vi "17O std simple.vi"(8 "error in":errorcluster) -> (0 "error out":errorcluster)   [LabVIEW 2016]
uses:
  controls/data control cluster.ctl
panel:
  out "transposed array":dbl[][](array[numeric])
  in  "number of sequence to combine":dbl=1.0
  out "Array":dbl[][](array[numeric])
  out "output cluster":T1
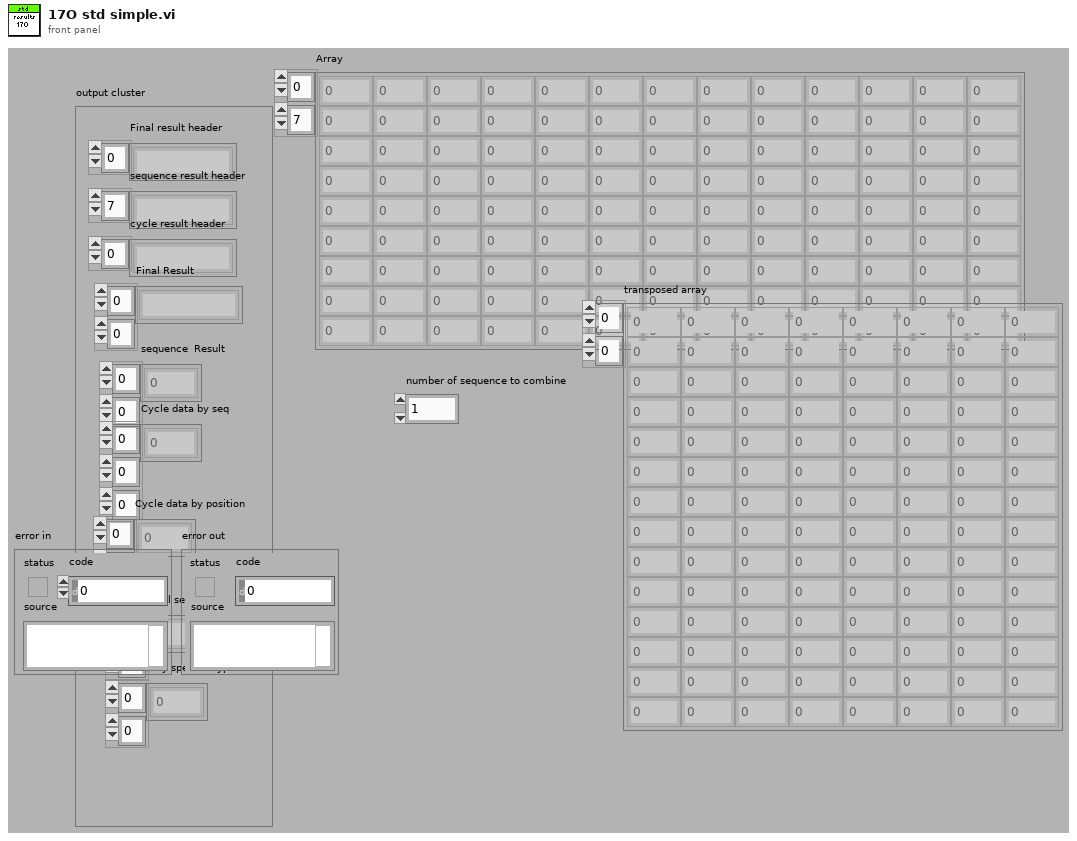
[diagram p1: front panel]
types:
  T1 = typedef "data control cluster.ctl" = cluster{"Final result header":string[], "sequence result header":string[], "cycle result header ":string[], "Final Result":string[][], "sequence  Result":dbl[][], "Cycle data by seq":dbl[][][], "Cycle data by position":dbl[][][], "Final seq  Result":dbl[][], "only specific type":dbl[][]}
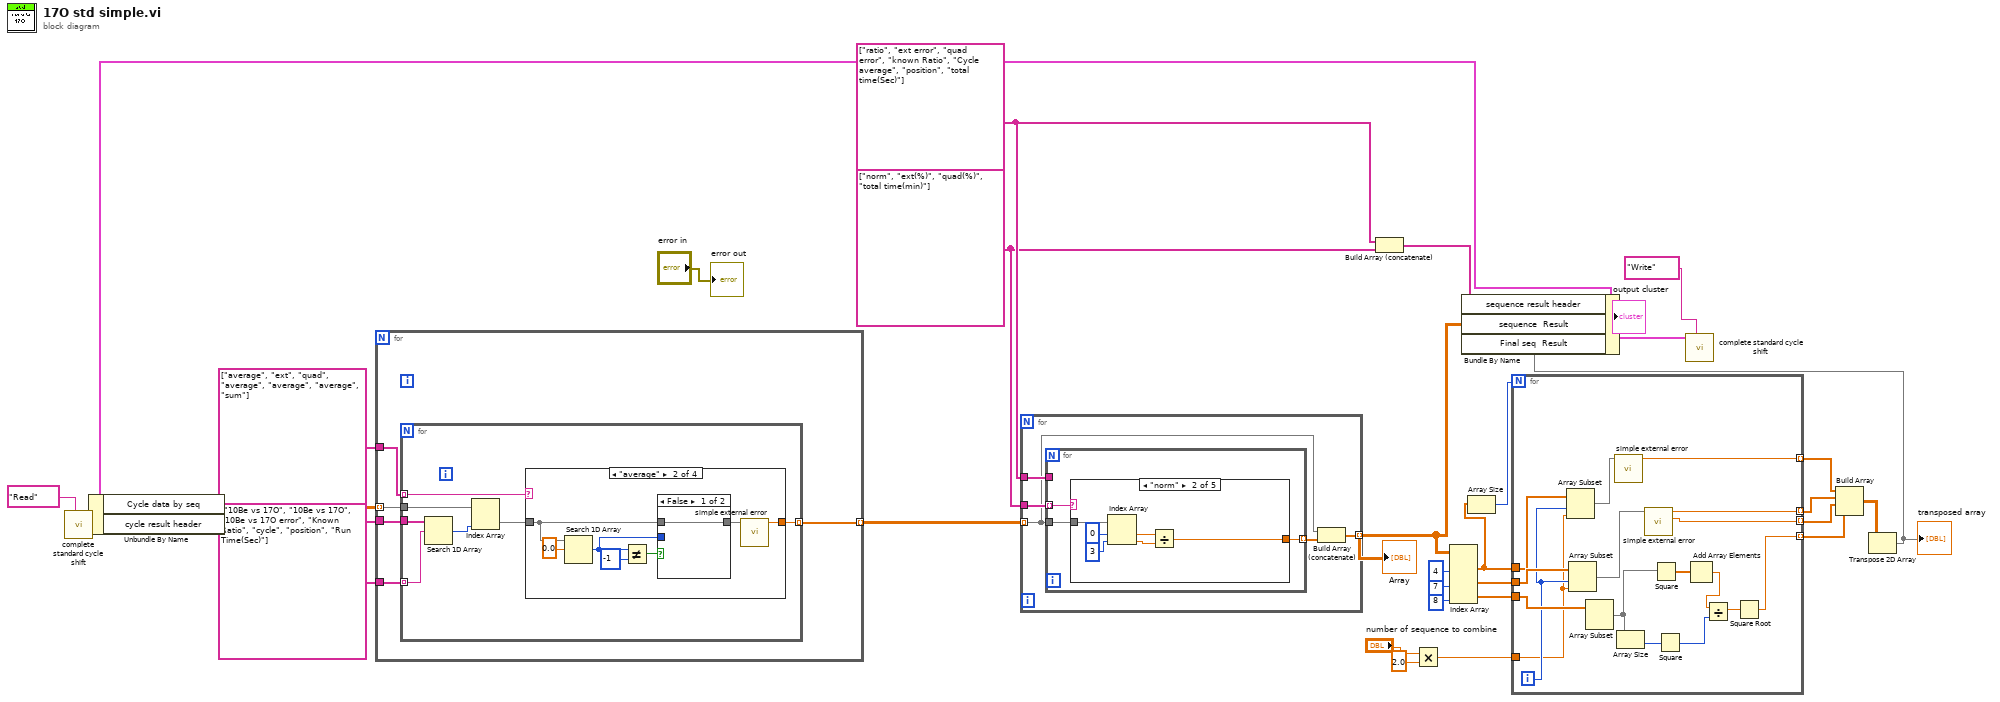
[diagram p0: block diagram]
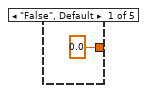
[diagram p2: hidden frame]
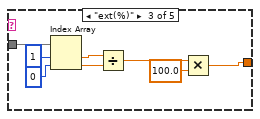
[diagram p3: hidden frame]
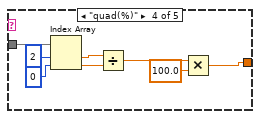
[diagram p4: hidden frame]
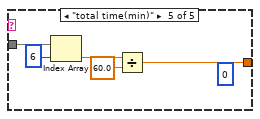
[diagram p5: hidden frame]
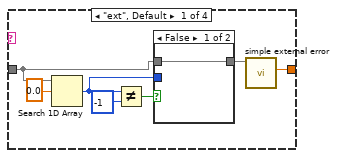
[diagram p6: hidden frame]
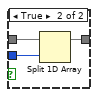
[diagram p7: hidden frame]
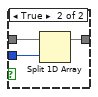
[diagram p8: hidden frame]
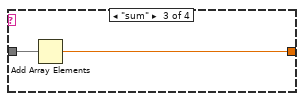
[diagram p9: hidden frame]
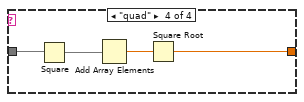
[diagram p10: hidden frame]
diagram:
  w25 = string[] ["ratio", "ext error", "quad error", "known Ratio", "Cycle average", "position", "total time(Sec)"]
  w24 = string[] ["norm", "ext(%)", "quad(%)", "total time(min)"]
  n1 = call "complete standard cycle shift.vi"("read write shift"="Read") -> ("DATA CLUSTER out"=w22:T1)  [unwired: 9 in, 1 out]
  n2 = Unbundle By Name(w22) -> ("Cycle data by seq"=w30:dbl[][][], "cycle result header"=w29:string[])
  n3 = for {
    tunnel: w30 -> [w33] mode=indexing
    tunnel: w29 -> [w35]
    tunnel: string[] ["10Be vs 17O", "10Be vs 17O", "10Be vs 17O error", "Known Ratio", "cycle", "position", "Run Time(Sec)"] -> [w34]
    tunnel: string[] ["average", "ext", "quad", "average", "average", "average", "sum"] -> [w32]
    tunnel: [w31] -> w26 mode=indexing
    n4 = for {
      tunnel: w35 -> [w42]
      tunnel: w34 -> [w41] mode=indexing
      tunnel: w33 -> [w40]
      tunnel: w32 -> [w39] mode=indexing
      tunnel: [w37] -> w31 mode=indexing
      n5 = Search 1D Array(1D array=w42, element=w41) -> (index of element=w36:i32)  [unwired: 1 in]
      n6 = Index Array(array=w40, index (col)=w36) -> (element=w38:dbl[])  [unwired: 1 in]
      n7 = case shown="\"average\"" w39 {
        tunnel: w38 -> [w47 w58 w66 w70]
        tunnel: [w49 w60 w65 w67] -> w37
        frame "ext", Default {
          n8 = Search 1D Array(1D array=w47, element=0.0) -> (index of element=w44:i32)  [unwired: 1 in]
          n9 = Not Equal?(x=w44, y=-1) -> (x != y?=w45:bool)
          n10 = case shown="False" w45 {
            tunnel: w44 -> [_ w53]
            tunnel: w47 -> [w50 w52]
            tunnel: [w50 w51] -> w46
            frame False {
            }
            frame True {
              n11 = Split 1D Array(array=w52, index=w53) -> (first subarray=w51:dbl[])  [unwired: 1 out]
            }
          }
          n12 = call "simple external error.vi"("cycle results"=w46) -> ("External error"=w49:dbl)  [unwired: 7 in, 3 out]
        }
        frame "average" {
          n13 = Search 1D Array(1D array=w58, element=0.0) -> (index of element=w55:i32)  [unwired: 1 in]
          n14 = Not Equal?(x=w55, y=-1) -> (x != y?=w56:bool)
          n15 = case shown="False" w56 {
            tunnel: w55 -> [_ w64]
            tunnel: w58 -> [w61 w63]
            tunnel: [w61 w62] -> w57
            frame False {
            }
            frame True {
              n16 = Split 1D Array(array=w63, index=w64) -> (first subarray=w62:dbl[])  [unwired: 1 out]
            }
          }
          n17 = call "simple external error.vi"("cycle results"=w57) -> ("Sequence result"=w60:dbl)  [unwired: 7 in, 3 out]
        }
        frame "sum" {
          n18 = Add Array Elements(numeric array=w66) -> (sum=w65:dbl)
        }
        frame "quad" {
          n19 = Square(x=w70) -> (x^2=w69:dbl[])
          n20 = Add Array Elements(numeric array=w69) -> (sum=w68:dbl)
          n21 = Square Root(x=w68) -> (sqrt(x)=w67:dbl)
        }
      }
    }
  }
  n22 = for {
    tunnel: w26 -> [w72] mode=indexing
    tunnel: w24 -> [w75]
    tunnel: w25 -> [w74]
    tunnel: [w71] -> w15 mode=indexing
    n23 = for {
      tunnel: w75 -> [w78] mode=indexing
      tunnel: w74 -> [_]
      tunnel: w72 -> [w77]
      tunnel: [w76] -> w73 mode=indexing
      n24 = case shown="\"norm\"" w78 {
        tunnel: w77 -> [_ w85 w93 w101 w106]
        tunnel: [0.0 w80 w86 w94 w102] -> w76
        frame "False", Default {
        }
        frame "norm" {
          n25 = Index Array(array=w85, index #1=0 ("index"), index #2=3 ("index")) -> (element #1=w81:dbl, element #2=w82:dbl)
          n26 = Divide(x=w81, y=w82) -> (x/y=w80:dbl)
        }
        frame "ext(%)" {
          n27 = Index Array(array=w93, index #1=1 ("index"), index #2=0 ("index")) -> (element #1=w89:dbl, element #2=w90:dbl)
          n28 = Divide(x=w89, y=w90) -> (x/y=w88:dbl)
          n29 = Multiply(x=w88, y=100.0) -> (x*y=w86:dbl)
        }
        frame "quad(%)" {
          n30 = Index Array(array=w101, index #1=2 ("index"), index #2=0 ("index")) -> (element #1=w97:dbl, element #2=w98:dbl)
          n31 = Divide(x=w97, y=w98) -> (x/y=w96:dbl)
          n32 = Multiply(x=w96, y=100.0) -> (x*y=w94:dbl)
        }
        frame "total time(min)" {
          (unwired) 0 ("index")
          n33 = Index Array(array=w106, index=6) -> (element=w104:dbl)
          n34 = Divide(x=w104, y=60.0) -> (x/y=w102:dbl)
        }
      }
    }
    n35 = Build Array (concatenate)(w72, w73) -> (w71:dbl[])
  }
  "Array" <- w15
  n36 = Build Array (concatenate)(w25, w24) -> (w23:string[])
  n37 = Multiply(x="number of sequence to combine", y=2.0) -> (x*y=w9:dbl)
  n38 = Index Array(array=w15, index (col) #1=4 ("disabled index (col)"), index (col) #2=7 ("index (col)"), index (col) #3=8 ("index (col)")) -> (element #1=w8:dbl[], element #2=w11:dbl[], element #3=w10:dbl[])  [unwired: 3 in]
  n39 = Array Size(array=w8) -> (size(s)=w7:i32)
  n40 = for {
    N: w7 -> [_]
    tunnel: w8 -> [w108]
    tunnel: w11 -> [w123]
    tunnel: w10 -> [w122]
    tunnel: w9 -> [w109]
    tunnel: [w120] -> w5 mode=indexing
    tunnel: [w119] -> w4 mode=indexing
    tunnel: [w112] -> w3 mode=indexing
    tunnel: [w111] -> w6 mode=indexing
    i -> [w110]
    n41 = Array Subset(array=w108, index=w110, length=w109) -> (w107:dbl[])
    n42 = Array Subset(array=w123, index=w110, length=w109) -> (w121:dbl[])
    n43 = Array Subset(array=w122) -> (w117:dbl[])  [unwired: 2 in]
    n44 = call "simple external error.vi"("cycle results"=w107) -> ("Sequence result"=w111:dbl)  [unwired: 7 in, 3 out]
    n45 = Array Size(array=w117) -> (size(s)=w118:i32)
    n46 = call "simple external error.vi"("cycle results"=w121) -> ("External error"=w119:dbl, "Sequence result"=w120:dbl)  [unwired: 7 in, 2 out]
    n47 = Square(x=w117) -> (x^2=w116:dbl[])
    n48 = Square(x=w118) -> (x^2=w115:i32)
    n49 = Add Array Elements(numeric array=w116) -> (sum=w114:dbl)
    n50 = Divide(x=w114, y=w115) -> (x/y=w113:dbl)
    n51 = Square Root(x=w113) -> (sqrt(x)=w112:dbl)
  }
  n52 = Build Array(w6, w5, w4, w3) -> (w2:dbl[][])
  n53 = Transpose 2D Array(2D array=w2) -> (transposed array=w1:dbl[][])
  "transposed array" <- w1
  n54 = Bundle By Name(cluster=w22, "sequence result header"=w23, "sequence  Result"=w15, "Final seq  Result"=w1) -> (w19:T1)
  "output cluster" <- w19
  n55 = call "complete standard cycle shift.vi"("read write shift"="Write", "DATA CLUSTER in"=w19) -> ()  [unwired: 8 in, 2 out]
  "error out" <- "error in"
